vi "Opposite Numeric Operation.vi"(1 "Operand 2":string, 2 "Operator":string, 3 "Operand 1":u64) -> (0 "Result":u64)   [LabVIEW 2020, in "AoC 2022.lvlib"]
uses:
  AoC 2022.lvlib
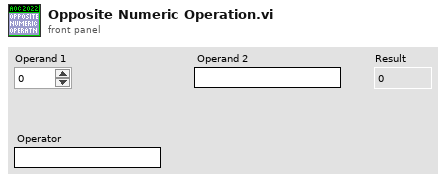
[diagram p1: front panel]
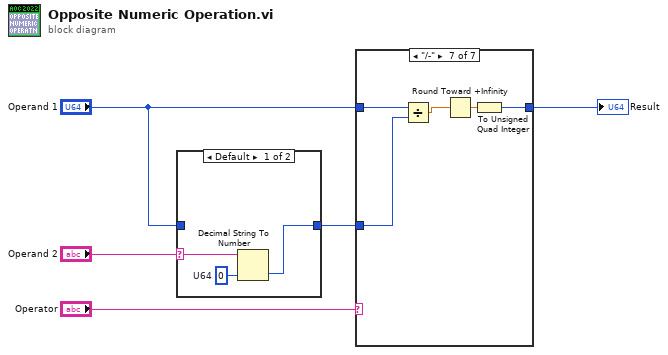
[diagram p0: block diagram]
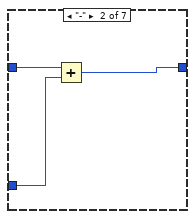
[diagram p4: hidden frame]
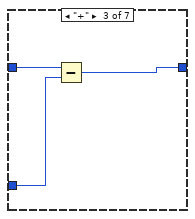
[diagram p5: hidden frame]
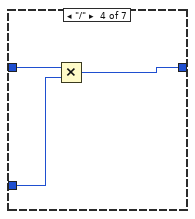
[diagram p6: hidden frame]
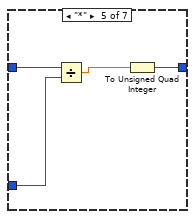
[diagram p7: hidden frame]
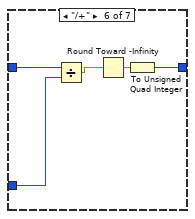
[diagram p8: hidden frame]
diagram:
  n1 = case shown="Default" "Operand 2" {
    selector: "Operand 2" -> [w8 _]
    tunnel: "Operand 1" -> [_ w9]
    tunnel: [w7 w9] -> w4
    frame Default {
      w6 = u64 0  # U64
      n2 = Decimal String To Number(string=w8, default (0L)=w6) -> (number=w7:u64)  [unwired: 1 in, 1 out]
    }
    frame "old" {
    }
  }
  n3 = case shown="\"/-\"" "Operator" {
    tunnel: "Operand 1" -> [w10 w13 w16 w19 w23 w28 w33]
    tunnel: w4 -> [_ w12 w15 w18 w22 w27 w32]
    tunnel: [w10 w11 w14 w17 w21 w24 w29] -> w5
    frame Default {
    }
    frame "-" {
      n4 = Add(x=w13, y=w12) -> (x+y=w11:u64)
    }
    frame "+" {
      n5 = Subtract(x=w16, y=w15) -> (x-y=w14:u64)
    }
    frame "/" {
      n6 = Multiply(x=w19, y=w18) -> (x*y=w17:u64)
    }
    frame "*" {
      n7 = Divide(x=w23, y=w22) -> (x/y=w20:dbl)
      n8 = To Unsigned Quad Integer(1:w20) -> (0:w21:u64)
    }
    frame "/+" {
      n9 = Divide(x=w28, y=w27) -> (x/y=w26:dbl)
      n10 = Round Toward -Infinity(1:w26) -> (0:w25:dbl)
      n11 = To Unsigned Quad Integer(1:w25) -> (0:w24:u64)
    }
    frame "/-" {
      n12 = Divide(x=w33, y=w32) -> (x/y=w31:dbl)
      n13 = Round Toward +Infinity(x=w31) -> (ceil(x): smallest int >= x=w30:dbl)
      n14 = To Unsigned Quad Integer(1:w30) -> (0:w29:u64)
    }
  }
  "Result" <- w5
